vi "PLC_OP10_Write.vi"(0 "S7 Connection in":T1, 5 "value change as error ?":bool, 11 "error in (no error)":errorcluster) -> (4 "S7 Connection out":T1, 15 "error out":errorcluster)   [LabVIEW 2017]
uses:
  <vilib>/DATA AHEAD/SP7/typedefs/S7 Connection.ctl
  <vilib>/DATA AHEAD/SP7/typedefs/PLC Type.ctl
  6203fae9-b88f-4171-836b-31210aefc1f5.vi
  Global/DATA LOG.vi
  <vilib>/DATA AHEAD/SP7/functions/write/write Dint array.vi
  Global/Global 1.vi
  <vilib>/DATA AHEAD/SP7/functions/write/writeString.vi
  <vilib>/DATA AHEAD/SP7/SP7.lvlib
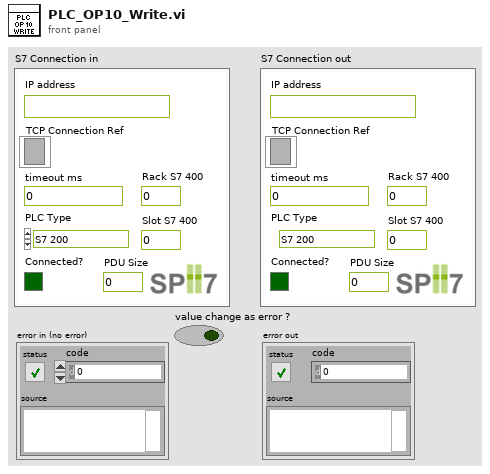
[diagram p1: front panel]
types:
  T1 = typedef "SP7.lvlib/S7 Connection.ctl" = cluster{"TCP Connection Ref":refnum<k5>, "IP address":string, "timeout ms":i32, "Connected?":bool, "PLC Type":T2, "Rack S7 400":u8, "Slot S7 400":u8, "PDU Size":u16, "connection semaphore":T3}
  T2 = typedef "SP7.lvlib/PLC Type.ctl" = enum16{"S7 200", "S7 300/400", "S7 1200", "S7 1500", "LOGO!8"}
  T3 = typedef "Semaphore RefNum" = refnum<k1>
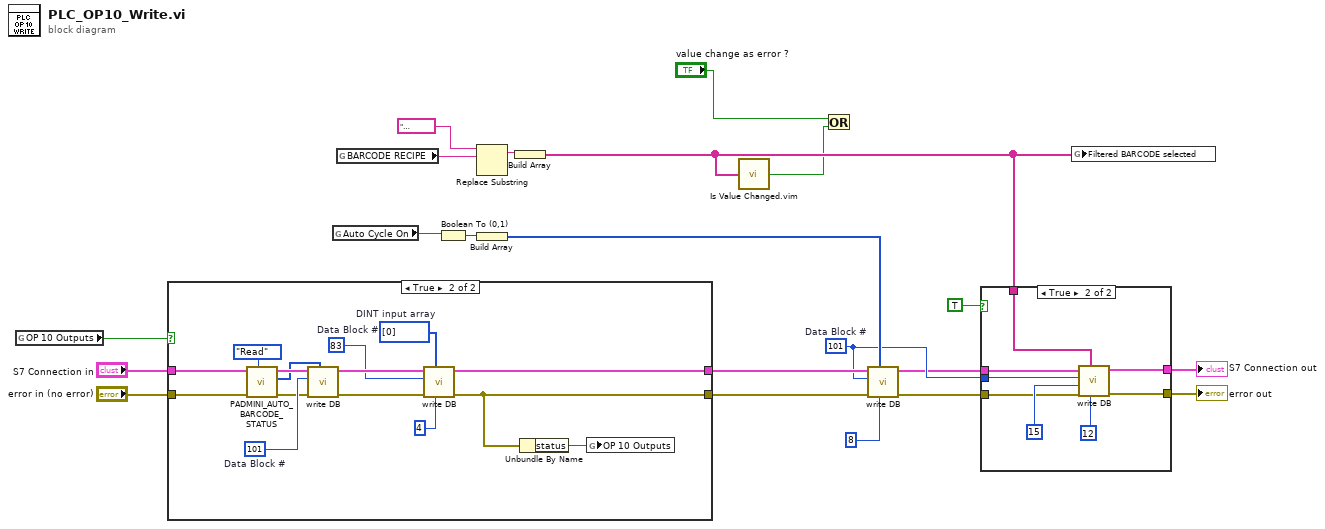
[diagram p0: block diagram]
diagram:
  w7 = u16 101  # Data Block #
  n1 = global read "DATA LOG.vi" "OP 10 Outputs"() -> (w14:bool)
  n2 = case shown="True" w14 {
    tunnel: "S7 Connection in" -> [w22 w36]
    tunnel: [w23 w25] -> w16
    tunnel: [w22 w29] -> w15
    tunnel: "error in (no error)" -> [w23 w33]
    frame False {
    }
    frame True {
      w26 = i32[] [0]  # DINT input array
      w28 = u16 83  # Data Block #
      w37 = u16 101  # Data Block #
      n3 = call "PADMINI_AUTO_BARCODE_STATUS.vi"("Enum"=enum16{"Read", "Write"}."Read", "error in (no error)"=w33) -> ("error out"=w32:errorcluster, "O/P"=w34:i32[])  [unwired: 8 in]
      n4 = call-poly <vilib>:"write DB.vi"("DINT input array"=w34, "error in (no error)"=w32, "Data Block #"=w37, "S7 Connection in"=w36) -> ("error out"=w31:errorcluster, "S7 Connection out"=w30:T1)  [unwired: 4 in, 2 out]
      n5 = call-poly <vilib>:"write DB.vi"("Item offset [byte]"=u32 4, "DINT input array"=w26, "error in (no error)"=w31, "Data Block #"=w28, "S7 Connection in"=w30) -> ("error out"=w25:errorcluster, "S7 Connection out"=w29:T1)  [unwired: 3 in, 2 out]
      n6 = Unbundle By Name(w25) -> ("status"=w24:bool)
      n7 = global write "DATA LOG.vi" "OP 10 Outputs"(w24) -> ()
    }
  }
  n8 = global read "DATA LOG.vi" "Auto Cycle On"() -> (w11:bool)
  n9 = global read "Global 1.vi" "BARCODE RECIPE"() -> (w20:string)
  n10 = Boolean To (0,1)(Boolean=w11) -> (0, 1=w10:i16)
  n11 = Replace Substring(4:w20, 5:"               ") -> (1:w21:string)  [unwired: 2 in, 1 out]
  n12 = Build Array(w10) -> (w8:i16[])
  n13 = Build Array(w21) -> (w9:string[])
  n14 = call "Is Value Changed.vim"("value"=w9) -> ("changed or first call?"=w2:bool)
  n15 = Or(x="value change as error ?", y=w2) -> ()  [unwired: 1 out]
  n16 = call-poly <vilib>:"write DB.vi"("Item offset [byte]"=u32 8, "DINT input array"=w8, "error in (no error)"=w16, "Data Block #"=w7, "S7 Connection in"=w15) -> ("error out"=w6:errorcluster, "S7 Connection out"=w4:T1)  [unwired: 3 in, 2 out]
  n17 = case shown="True" TRUE {
    tunnel: [w39 w47] -> w18
    tunnel: [w38 w46] -> w17
    tunnel: w9 -> [_ w45]
    tunnel: w7 -> [_ w42]
    tunnel: w6 -> [w39 w41]
    tunnel: w4 -> [w38 w40]
    frame False {
    }
    frame True {
      n18 = call-poly <vilib>:"write DB.vi"("Item offset [byte]"=u32 12, "Input STRINGS"=w45, "error in (no error)"=w41, "String length reserved in DB (default=254)"=u16 15, "Data Block #"=w42, "S7 Connection in"=w40) -> ("error out"=w47:errorcluster, "S7 Connection out"=w46:T1)  [unwired: 2 in, 2 out]
    }
  }
  "error out" <- w18
  "S7 Connection out" <- w17
  n19 = global write "Global 1.vi" "Filtered BARCODE selected"(w9) -> ()
